vi "Async Configuration.vi"(8 "error in":errorcluster, 11 "Data Cluster in":T1 {"Async serial Configuration Cluster"."Minor Frame Count" min=5 max=8 step=1}) -> (0 "error out":errorcluster, 2 "File out":refnum<file>, 3 "Data Cluster out":T1 {"Async serial Configuration Cluster"."Minor Frame Count" min=5 max=8 step=1})   [LabVIEW 2024]
uses:
  Controls/Async Serial State Machine Data Cluster.ctl
  <vilib>/Modbus/master/Modbus Master.lvclass
  Controls/Async Serial Command Q Cluster.ctl
  Controls/Async Serial Configuration Cluster.ctl
  Controls/Async Frame Info Cluster.ctl
  Controls/Async Message Info Cluster.ctl
  Main Engine/Controls/Main Engine JSON Command State.ctl
  TCP Engine/Controls/TCP Engine Serial Interupt Cluster.ctl
  Controls/Async Sensor Type.ctl
  Main Engine/Controls/Main Engine Config Confirmation Cluster.ctl
  <vilib>/Instr/_visa.llb/VISA Configure Serial Port (Instr).vi
  <vilib>/Modbus/master/Create Master Instance (Serial).vi
  TCP Engine/TCP Engine.lvlib
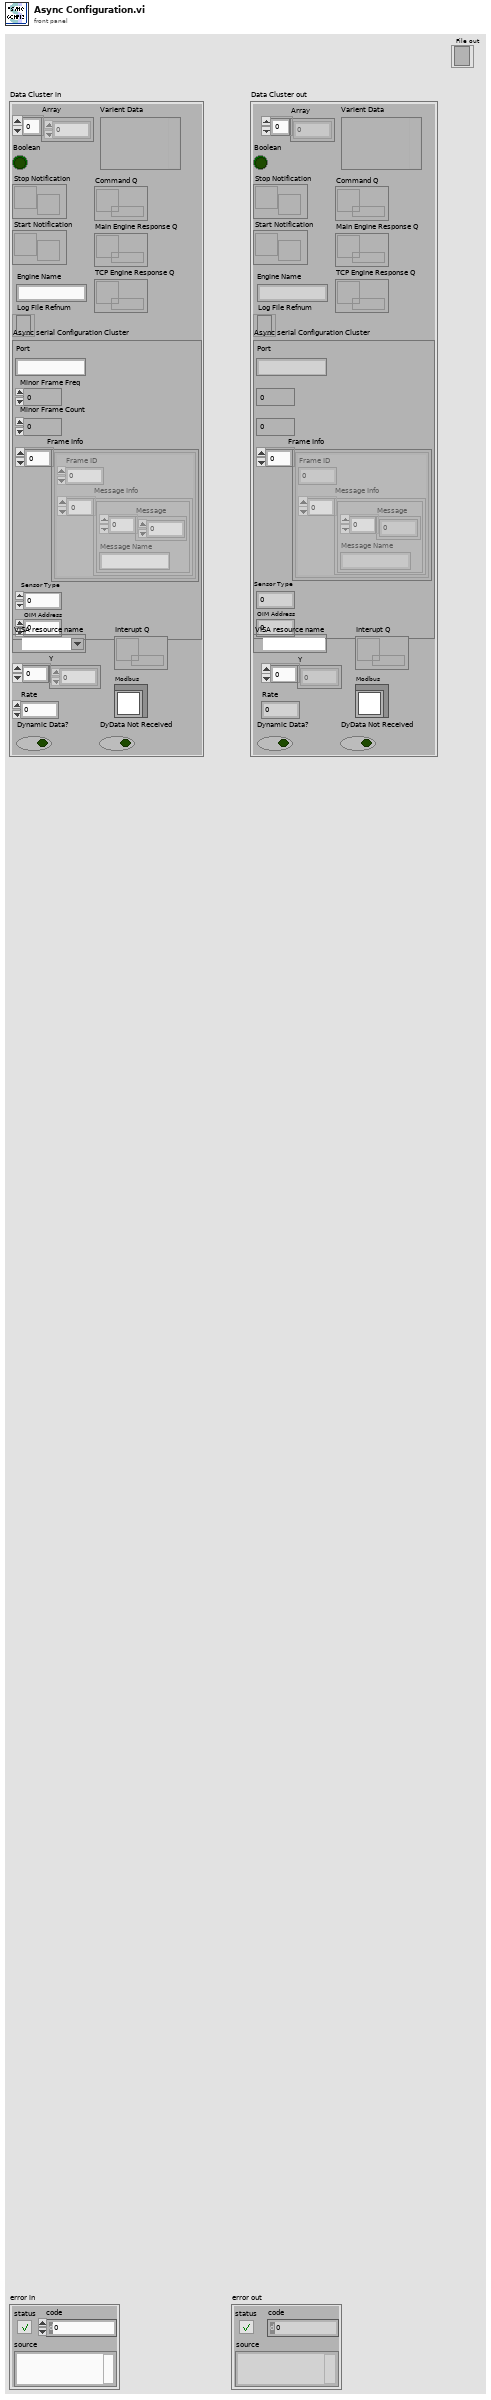
[diagram p1: front panel]
types:
  T1 = typedef "Async Serial State Machine Data Cluster.ctl" = cluster{"Array":dbl[], "Boolean":bool, "Varient Data":variant, "Stop Notification":refnum<notifier>, "Start Notification":refnum<notifier>, "Command Q":refnum<queue>, "Main Engine Response Q":refnum<queue>, "TCP Engine Response Q":refnum<queue>, "Engine Name":string, "Log File Refnum":refnum<file>, "Async serial Configuration Cluster":T2, "VISA resource name":refnum<visa-resource-name>, "Y":dbl[], "Rate":i32, "Dynamic Data?":bool, "DyData Not Received":bool, "Interupt Q":refnum<queue>, "Modbus":refnum<class "Modbus Master.lvclass">}
  T2 = typedef "Async Serial Configuration Cluster.ctl" = cluster{"Port":string, "Minor Frame Freq":u16, "Minor Frame Count":u16, "Frame Info":T3[], "Sensor Type":u16, "OIM Address":u16}
  T3 = typedef "Async Frame Info Cluster.ctl" = cluster{"Frame ID":u16, "Message Info":T4[]}
  T4 = typedef "Async Message Info Cluster.ctl" = cluster{"Message":u8[], "Message Name":string}
  T5 = typedef "Async Sensor Type.ctl" = enum16{"Camera", "INS", "Pri BMS", "Aux BMS", "Depth Sensor", "Altimeter", "OIM", "Thruster", "Acoustic Modem", "LED"}
  T6 = typedef "Main Engine Config Confirmation Cluster.ctl" = cluster{"Command":string, "Interface":string, "Status":string, "Board":string}
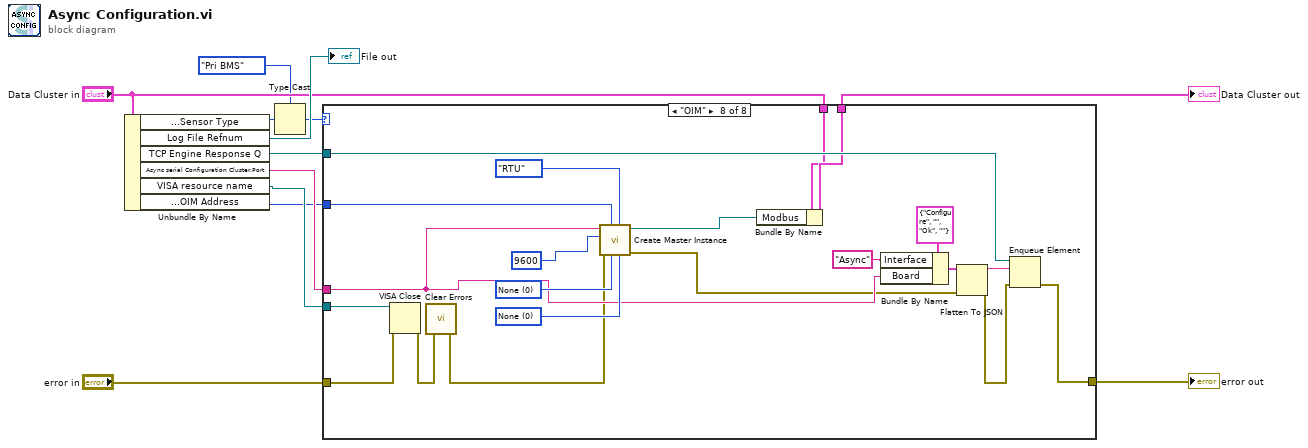
[diagram p0: block diagram]
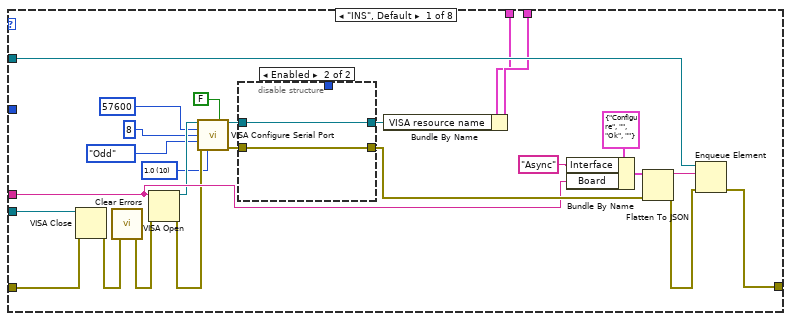
[diagram p2: hidden frame]
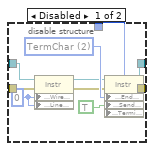
[diagram p3: hidden frame]
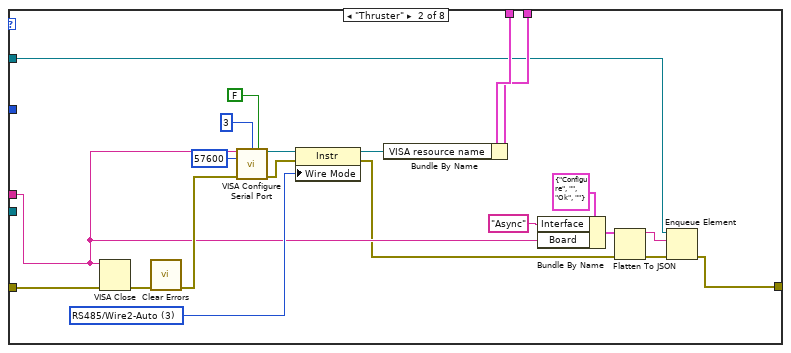
[diagram p4: hidden frame]
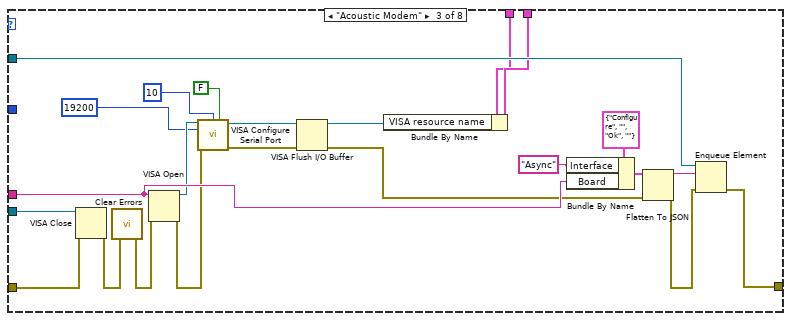
[diagram p5: hidden frame]
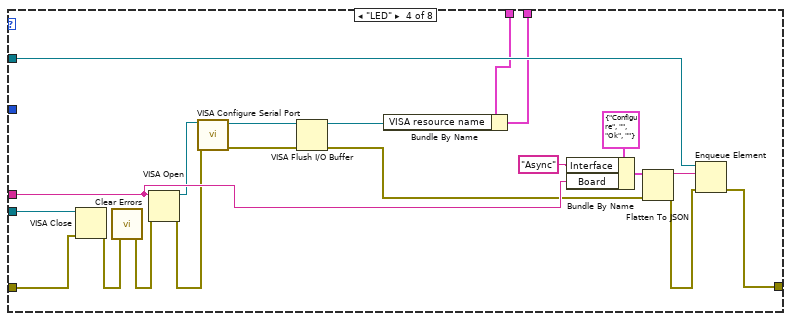
[diagram p6: hidden frame]
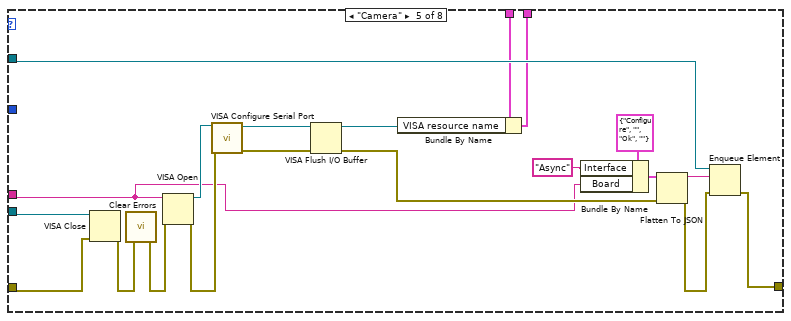
[diagram p7: hidden frame]
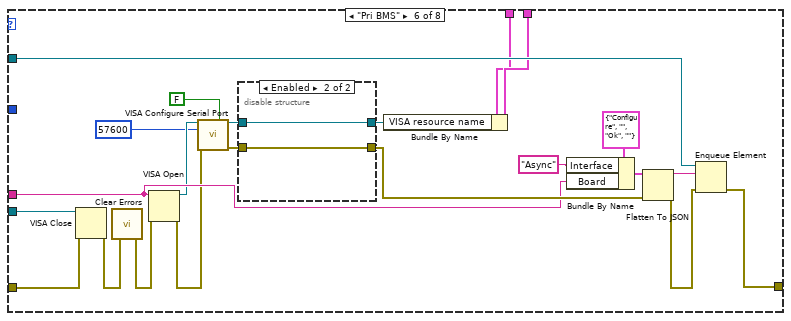
[diagram p8: hidden frame]
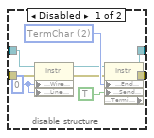
[diagram p9: hidden frame]
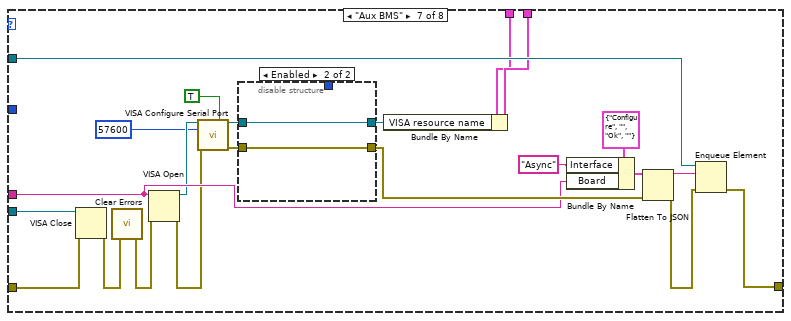
[diagram p10: hidden frame]
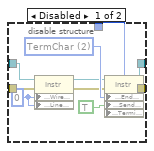
[diagram p11: hidden frame]
diagram:
  n1 = Unbundle By Name("Data Cluster in") -> ("Async serial Configuration Cluster.Sensor Type"=w6:u16, "Log File Refnum"=→"File out":refnum<file>, "TCP Engine Response Q"=w11:refnum<queue>, "Async serial Configuration Cluster.Port"=w3:string, "VISA resource name"=w2:refnum<visa-resource-name>, "Async serial Configuration Cluster.OIM Address"=w1:u16)
  n2 = Type Cast(type=Async_Sensor_Type."Pri BMS" ("Sensor Type"), x=w6) -> (*(type *) &x=w5:T5)
  n3 = case shown="\"OIM\"" w5 {
    tunnel: w3 -> [w33 w57 w93 w113 w118 w151 w185 w206]
    tunnel: w11 -> [w32 w52 w92 w112 w117 w150 w184 w222]
    tunnel: [w31 w50 w91 w111 w114 w149 w183 w221] -> w10
    tunnel: "error in" -> [w25 w70 w85 w105 w120 w143 w177 w215]
    tunnel: w2 -> [w22 _ w82 w102 w119 w140 w174 w213]
    tunnel: [w21 w60 w81 w101 w115 w139 w173 w212] -> w8
    tunnel: "Data Cluster in" -> [w20 w62 w80 w100 w116 w138 w172 w211]
    tunnel: w1 -> [_ _ _ _ _ _ _ w202]
    frame "INS", Default {
      w13 = u16 10 items=["1.0"=10, "1.5"=15, "2.0"=20] ("stop bits (10: 1 bit)")
      n4 = VISA Close(VISA resource name=w22, error in (no error)=w25) -> (error out=w23:errorcluster)
      n5 = call <vilib>:"Clear Errors.vi"("error in (no error)"=w23) -> ("error out"=w24:errorcluster)  [unwired: 5 in, 1 out]
      n6 = VISA Open(error in (no error)=w24, VISA resource name=w33) -> (VISA resource name=w18:refnum<visa-resource-name>, error out=w19:errorcluster)  [unwired: 3 in]
      n7 = call-poly "VISA Configure Serial Port"("VISA resource name"=w18, "Enable Termination\nChar (T)"=FALSE ("Enable Termination\nChar (T)"), "baud rate (9600)"=u32 57600, "data bits (8)"=u16 8, "parity (0:none)"=enum16{"None", "Odd", "Even", "Mark", "Space"}."Odd", "error in (no error)"=w19, "stop bits (10: 1 bit)"=w13) -> ("VISA resource name out"=w34:refnum<visa-resource-name>, "error out"=w36:errorcluster)  [unwired: 7 in]
      n8 = disable-structure shown="Enabled" {
        disable-tunnel: _ -> [w45 _]
        disable-tunnel: w34 -> [w42 w49]
        disable-tunnel: [w41 w49] -> w35
        disable-tunnel: w36 -> [w40 w48]
        disable-tunnel: [w39 w48] -> w37
        frame Disabled {
          w38 = i16 0 ("0, 2")
          w47 = u16 2 items=["None", "LastBit", "TermChar", "Break"] ("Serial Settings:Serial End Mode for Writes")
          n9 = property class="Instr"(reference=w42, error in=w40, "Serial Settings:Wire Mode"=w38, "Serial Settings:Modem Line Settings:Line DTR State"=w38) -> (reference out=w43:refnum<visa-resource-name>, error out=w44:errorcluster)
          n10 = property class="Instr"(reference=w43, error in=w44, "Serial Settings:End Mode for Writes"=w47, "Message Based Settings:Send End Enable"=TRUE, "Message Based Settings:Termination Character"=w45) -> (reference out=w41:refnum<visa-resource-name>, error out=w39:errorcluster)
        }
        frame Enabled {
        }
      }
      n11 = Bundle By Name(cluster=w20, "VISA resource name"=w35) -> (w21:T1)
      n12 = Bundle By Name(cluster=T6 {"Command"="Configure", "Interface"="", "Status"="Ok", "Board"=""}, "Interface"="Async" ("SubCmd"), "Board"=w33) -> (w26:T6)
      n13 = Flatten To JSON(anything=w26, error in (no error)=w37) -> (JSON string=w27:string, 11:w30:errorcluster)  [unwired: 1 in]
      n14 = Enqueue Element(queue=w32, element=w27, error in (no error)=w30) -> (error out=w31:errorcluster)  [unwired: 1 in, 2 out]
    }
    frame "Thruster" {
      w63 = i16 3 items=["Unknown"=-1, "RS485/Wire4"=0, "RS485/Wire2-EchoDTR"=1, "RS485/Wire2-CtrlDTR"=2, "RS485/Wire2-Auto"=3, "RS232/DTE"=128, "RS232/DCE"=129, "RS232/Auto"=130] ("Serial Settings:Wire Mode")
      n15 = VISA Close(VISA resource name=w57, error in (no error)=w70) -> (error out=w69:errorcluster)
      n16 = call <vilib>:"Clear Errors.vi"("error in (no error)"=w69) -> ("error out"=w68:errorcluster)  [unwired: 5 in, 1 out]
      n17 = call-poly "VISA Configure Serial Port"("VISA resource name"=w57, "termination char\n(0xA = '\\n' = LF)"=u8 3 ("termination char\n(0xA = '\\n' = LF)"), "Enable Termination\nChar (T)"=FALSE ("Enable Termination\nChar (T)"), "baud rate (9600)"=u32 57600, "error in (no error)"=w68) -> ("VISA resource name out"=w64:refnum<visa-resource-name>, "error out"=w56:errorcluster)  [unwired: 9 in]
      n18 = property class="Instr"(reference=w64, error in=w56, "Wire Mode"=w63) -> (reference out=w61:refnum<visa-resource-name>, error out=w54:errorcluster)
      n19 = Bundle By Name(cluster=w62, "VISA resource name"=w61) -> (w60:T1)
      n20 = Bundle By Name(cluster=T6 {"Command"="Configure", "Interface"="", "Status"="Ok", "Board"=""} ("Config Confirmation"), "Interface"="Async", "Board"=w57) -> (w55:T6)
      n21 = Flatten To JSON(anything=w55, error in (no error)=w54) -> (JSON string=w51:string, 11:w53:errorcluster)  [unwired: 1 in]
      n22 = Enqueue Element(queue=w52, element=w51, error in (no error)=w53) -> (error out=w50:errorcluster)  [unwired: 1 in, 2 out]
    }
    frame "Acoustic Modem" {
      n23 = VISA Close(VISA resource name=w82, error in (no error)=w85) -> (error out=w83:errorcluster)
      n24 = call <vilib>:"Clear Errors.vi"("error in (no error)"=w83) -> ("error out"=w84:errorcluster)  [unwired: 5 in, 1 out]
      n25 = VISA Open(error in (no error)=w84, VISA resource name=w93) -> (VISA resource name=w78:refnum<visa-resource-name>, error out=w79:errorcluster)  [unwired: 3 in]
      n26 = call-poly "VISA Configure Serial Port"("VISA resource name"=w78, "termination char\n(0xA = '\\n' = LF)"=u8 10 ("termination char\n(0xA = '\\n' = LF)"), "Enable Termination\nChar (T)"=FALSE ("Enable Termination\nChar (T)"), "baud rate (9600)"=u32 19200, "error in (no error)"=w79) -> ("VISA resource name out"=w72:refnum<visa-resource-name>, "error out"=w74:errorcluster)  [unwired: 9 in]
      n27 = VISA Flush I/O Buffer(VISA resource name=w72, error in (no error)=w74) -> (VISA resource name out=w71:refnum<visa-resource-name>, error out=w73:errorcluster)  [unwired: 1 in]
      n28 = Bundle By Name(cluster=w80, "VISA resource name"=w71) -> (w81:T1)
      n29 = Bundle By Name(cluster=T6 {"Command"="Configure", "Interface"="", "Status"="Ok", "Board"=""}, "Interface"="Async" ("SubCmd"), "Board"=w93) -> (w86:T6)
      n30 = Flatten To JSON(anything=w86, error in (no error)=w73) -> (JSON string=w87:string, 11:w90:errorcluster)  [unwired: 1 in]
      n31 = Enqueue Element(queue=w92, element=w87, error in (no error)=w90) -> (error out=w91:errorcluster)  [unwired: 1 in, 2 out]
    }
    frame "LED" {
      n32 = VISA Close(VISA resource name=w102, error in (no error)=w105) -> (error out=w103:errorcluster)
      n33 = call <vilib>:"Clear Errors.vi"("error in (no error)"=w103) -> ("error out"=w104:errorcluster)  [unwired: 5 in, 1 out]
      n34 = VISA Open(error in (no error)=w104, VISA resource name=w113) -> (VISA resource name=w98:refnum<visa-resource-name>, error out=w99:errorcluster)  [unwired: 3 in]
      n35 = call-poly "VISA Configure Serial Port"("VISA resource name"=w98, "error in (no error)"=w99) -> ("VISA resource name out"=w95:refnum<visa-resource-name>, "error out"=w97:errorcluster)  [unwired: 12 in]
      n36 = VISA Flush I/O Buffer(VISA resource name=w95, error in (no error)=w97) -> (VISA resource name out=w94:refnum<visa-resource-name>, error out=w96:errorcluster)  [unwired: 1 in]
      n37 = Bundle By Name(cluster=w100, "VISA resource name"=w94) -> (w101:T1)
      n38 = Bundle By Name(cluster=T6 {"Command"="Configure", "Interface"="", "Status"="Ok", "Board"=""}, "Interface"="Async" ("SubCmd"), "Board"=w113) -> (w106:T6)
      n39 = Flatten To JSON(anything=w106, error in (no error)=w96) -> (JSON string=w107:string, 11:w110:errorcluster)  [unwired: 1 in]
      n40 = Enqueue Element(queue=w112, element=w107, error in (no error)=w110) -> (error out=w111:errorcluster)  [unwired: 1 in, 2 out]
    }
    frame "Camera" {
      n41 = VISA Close(VISA resource name=w119, error in (no error)=w120) -> (error out=w127:errorcluster)
      n42 = call <vilib>:"Clear Errors.vi"("error in (no error)"=w127) -> ("error out"=w128:errorcluster)  [unwired: 5 in, 1 out]
      n43 = VISA Open(error in (no error)=w128, VISA resource name=w118) -> (VISA resource name=w125:refnum<visa-resource-name>, error out=w126:errorcluster)  [unwired: 3 in]
      n44 = call-poly "VISA Configure Serial Port"("VISA resource name"=w125, "error in (no error)"=w126) -> ("VISA resource name out"=w122:refnum<visa-resource-name>, "error out"=w124:errorcluster)  [unwired: 12 in]
      n45 = VISA Flush I/O Buffer(VISA resource name=w122, error in (no error)=w124) -> (VISA resource name out=w121:refnum<visa-resource-name>, error out=w123:errorcluster)  [unwired: 1 in]
      n46 = Bundle By Name(cluster=w116, "VISA resource name"=w121) -> (w115:T1)
      n47 = Bundle By Name(cluster=T6 {"Command"="Configure", "Interface"="", "Status"="Ok", "Board"=""}, "Interface"="Async" ("SubCmd"), "Board"=w118) -> (w129:T6)
      n48 = Flatten To JSON(anything=w129, error in (no error)=w123) -> (JSON string=w130:string, 11:w133:errorcluster)  [unwired: 1 in]
      n49 = Enqueue Element(queue=w117, element=w130, error in (no error)=w133) -> (error out=w114:errorcluster)  [unwired: 1 in, 2 out]
    }
    frame "Pri BMS" {
      n50 = VISA Close(VISA resource name=w140, error in (no error)=w143) -> (error out=w141:errorcluster)
      n51 = call <vilib>:"Clear Errors.vi"("error in (no error)"=w141) -> ("error out"=w142:errorcluster)  [unwired: 5 in, 1 out]
      n52 = VISA Open(error in (no error)=w142, VISA resource name=w151) -> (VISA resource name=w136:refnum<visa-resource-name>, error out=w137:errorcluster)  [unwired: 3 in]
      n53 = call-poly "VISA Configure Serial Port"("VISA resource name"=w136, "Enable Termination\nChar (T)"=FALSE ("Enable Termination\nChar (T)"), "baud rate (9600)"=u32 57600, "error in (no error)"=w137) -> ("VISA resource name out"=w152:refnum<visa-resource-name>, "error out"=w154:errorcluster)  [unwired: 10 in]
      n54 = disable-structure shown="Enabled" {
        disable-tunnel: w152 -> [w160 w167]
        disable-tunnel: [w159 w167] -> w153
        disable-tunnel: w154 -> [w158 w166]
        disable-tunnel: [w157 w166] -> w155
        frame Disabled {
          w156 = i16 0 ("0, 2")
          w165 = u16 2 items=["None", "LastBit", "TermChar", "Break"] ("Serial Settings:Serial End Mode for Writes")
          n55 = property class="Instr"(reference=w160, error in=w158, "Serial Settings:Wire Mode"=w156, "Serial Settings:Modem Line Settings:Line DTR State"=w156) -> (reference out=w161:refnum<visa-resource-name>, error out=w162:errorcluster)
          n56 = property class="Instr"(reference=w161, error in=w162, "Serial Settings:End Mode for Writes"=w165, "Message Based Settings:Send End Enable"=TRUE) -> (reference out=w159:refnum<visa-resource-name>, error out=w157:errorcluster, "Message Based Settings:Termination Character"=w163:u8)
        }
        frame Enabled {
        }
      }
      n57 = Bundle By Name(cluster=w138, "VISA resource name"=w153) -> (w139:T1)
      n58 = Bundle By Name(cluster=T6 {"Command"="Configure", "Interface"="", "Status"="Ok", "Board"=""}, "Interface"="Async" ("SubCmd"), "Board"=w151) -> (w144:T6)
      n59 = Flatten To JSON(anything=w144, error in (no error)=w155) -> (JSON string=w145:string, 11:w148:errorcluster)  [unwired: 1 in]
      n60 = Enqueue Element(queue=w150, element=w145, error in (no error)=w148) -> (error out=w149:errorcluster)  [unwired: 1 in, 2 out]
    }
    frame "Aux BMS" {
      n61 = VISA Close(VISA resource name=w174, error in (no error)=w177) -> (error out=w175:errorcluster)
      n62 = call <vilib>:"Clear Errors.vi"("error in (no error)"=w175) -> ("error out"=w176:errorcluster)  [unwired: 5 in, 1 out]
      n63 = VISA Open(error in (no error)=w176, VISA resource name=w185) -> (VISA resource name=w170:refnum<visa-resource-name>, error out=w171:errorcluster)  [unwired: 3 in]
      n64 = call-poly "VISA Configure Serial Port"("VISA resource name"=w170, "Enable Termination\nChar (T)"=TRUE ("Enable Termination\nChar (T)"), "baud rate (9600)"=u32 57600, "error in (no error)"=w171) -> ("VISA resource name out"=w186:refnum<visa-resource-name>, "error out"=w188:errorcluster)  [unwired: 10 in]
      n65 = disable-structure shown="Enabled" {
        disable-tunnel: _ -> [w197 _]
        disable-tunnel: w186 -> [w194 w201]
        disable-tunnel: [w193 w201] -> w187
        disable-tunnel: w188 -> [w192 w200]
        disable-tunnel: [w191 w200] -> w189
        frame Disabled {
          w190 = i16 0 ("0, 2")
          w199 = u16 2 items=["None", "LastBit", "TermChar", "Break"] ("Serial Settings:Serial End Mode for Writes")
          n66 = property class="Instr"(reference=w194, error in=w192, "Serial Settings:Wire Mode"=w190, "Serial Settings:Modem Line Settings:Line DTR State"=w190) -> (reference out=w195:refnum<visa-resource-name>, error out=w196:errorcluster)
          n67 = property class="Instr"(reference=w195, error in=w196, "Serial Settings:End Mode for Writes"=w199, "Message Based Settings:Send End Enable"=TRUE, "Message Based Settings:Termination Character"=w197) -> (reference out=w193:refnum<visa-resource-name>, error out=w191:errorcluster)
        }
        frame Enabled {
        }
      }
      n68 = Bundle By Name(cluster=w172, "VISA resource name"=w187) -> (w173:T1)
      n69 = Bundle By Name(cluster=T6 {"Command"="Configure", "Interface"="", "Status"="Ok", "Board"=""}, "Interface"="Async" ("SubCmd"), "Board"=w185) -> (w178:T6)
      n70 = Flatten To JSON(anything=w178, error in (no error)=w189) -> (JSON string=w179:string, 11:w182:errorcluster)  [unwired: 1 in]
      n71 = Enqueue Element(queue=w184, element=w179, error in (no error)=w182) -> (error out=w183:errorcluster)  [unwired: 1 in, 2 out]
    }
    frame "OIM" {
      w210 = u16 0 items=["None", "XON/XOFF", "RTS/CTS", "XON/XOFF & RTS/CTS", "DTR/DSR", "XON/XOFF & DTR/DSR"] ("flow control (None)")
      w208 = u16 0 items=["None", "Odd", "Even"] ("parity (Even)")
      n72 = VISA Close(VISA resource name=w213, error in (no error)=w215) -> (error out=w214:errorcluster)
      n73 = call <vilib>:"Clear Errors.vi"("error in (no error)"=w214) -> ("error out"=w205:errorcluster)  [unwired: 5 in, 1 out]
      n74 = call-poly <vilib>:"Create Master Instance.vi"("flow control (None)"=w210, "serial type"=enum16{"RTU", "ASCII"}."RTU", "parity (Even)"=w208, "unit ID"=w202, "error in (no error)"=w205, "baud rate (9600)"=u32 9600, "VISA resource name"=w206) -> ("error out"=w204:errorcluster, "serial master instance"=w203:refnum<class "Modbus Master.lvclass">)  [unwired: 3 in]
      n75 = Bundle By Name(cluster=w211, "Modbus"=w203) -> (w212:T1)
      n76 = Bundle By Name(cluster=T6 {"Command"="Configure", "Interface"="", "Status"="Ok", "Board"=""}, "Interface"="Async" ("SubCmd"), "Board"=w206) -> (w216:T6)
      n77 = Flatten To JSON(anything=w216, error in (no error)=w204) -> (JSON string=w217:string, 11:w220:errorcluster)  [unwired: 1 in]
      n78 = Enqueue Element(queue=w222, element=w217, error in (no error)=w220) -> (error out=w221:errorcluster)  [unwired: 1 in, 2 out]
    }
  }
  "error out" <- w10
  "Data Cluster out" <- w8
